vi "编码器线性位置测量_连续.vi"() -> ()   [LabVIEW 2013]
uses:
  <userlib>/ArtDAQ/_SubVI/ArtDAQ_CreateCILinEncoderChan.vi
  <userlib>/ArtDAQ/_SubVI/ArtDAQ_CfgSampClkTiming.vi
  <userlib>/ArtDAQ/_SubVI/ArtDAQ_Read Counter DBL NSamp.vi
panel:
  out "数据(米)":dbl[](array[numeric])
  in  "时钟源":string="/Dev1/PFI0"
  in  "每通道点数":i32=100
  in  "采样频率":dbl=1000.0 caption="采样速率" format="%0.6f"
  in  "Z索引相位":i32(ring)=10040 items=["A高B高"=10040, "A高B低"=10041, "A低B高"=10042, "A低B低"=10043]
  in  "解码类型":i32(ring)=10090 items=["X1"=10090, "X2"=10091, "X4"=10092, "TwoPulse"=10313]
  in  "脉冲间隔":dbl=0.0001
  in  "初始位置":dbl
  in  "Z索引值":dbl
  in  "启用Z索引":bool
  in  "Stop":bool
  in  "计数器":string="Dev1/ctr0"
  out "错误输出":errorcluster
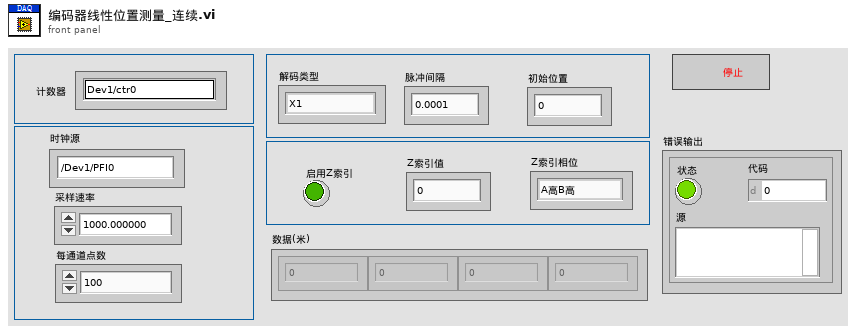
[diagram p1: front panel]
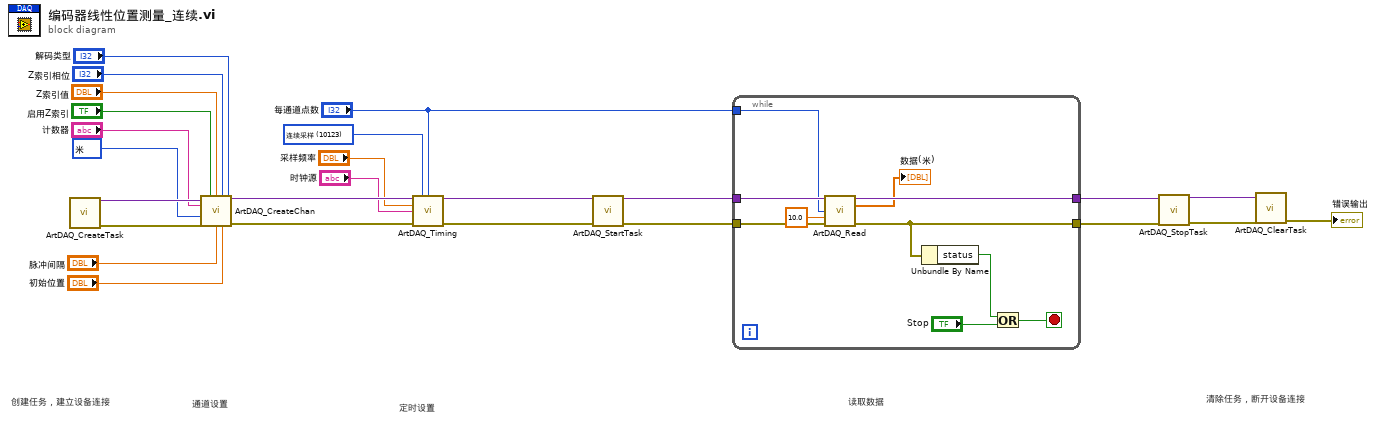
[diagram p0: block diagram]
diagram:
  w2 = 10123 items=["有限点采样"=10178, "连续采样"=10123] ("SampleMode")
  w11 = 10219 items=["米"=10219, "英寸"=10379, "时钟滴答"=10304, "来自自定义换算"=10065] ("单位")
  # "定时设置"
  # "清除任务，断开设备连接"
  # "读取数据"
  # "通道设置"
  # "创建任务，建立设备连接"
  n1 = call <userlib>:"ArtDAQ_CreateTask.vi"() -> ("任务句柄"=w25:variant, "错误输出"=w24:errorcluster)  [unwired: 14 in]
  n2 = call-poly <userlib>:"ArtDAQ_CreateChan.vi"("任务句柄"=w25, "启用Z索引"="启用Z索引", "Z索引值"="Z索引值", "Z索引相位"="Z索引相位", "计数器"="计数器", "解码类型"="解码类型", "单位"=w11, "错误输入"=w24, "脉冲间隔"="脉冲间隔", "初始位置"="初始位置") -> ("任务句柄"=w8:variant, "错误输出"=w5:errorcluster)  [unwired: 4 in]
  n3 = call-poly <userlib>:"ArtDAQ_Timing.vi"("任务句柄"=w8, "采样模式"=w2, "每通道采样数"="每通道点数", "采样率"="采样频率", "源"="时钟源", "错误输入"=w5) -> ("任务句柄"=w7:variant, "错误输出"=w6:errorcluster)  [unwired: 8 in]
  n4 = call <userlib>:"ArtDAQ_StartTask.vi"("任务句柄"=w7, "错误输入"=w6) -> ("任务句柄"=w14:variant, "错误输出"=w13:errorcluster)  [unwired: 12 in]
  n5 = while {
    tunnel: [w35] -> w22
    tunnel: [w34] -> w20
    tunnel: w14 -> [w33]
    tunnel: w13 -> [w32]
    tunnel: "每通道点数" -> [w26]
    stop <- w28 stop-if-true
    n6 = call-poly <userlib>:"ArtDAQ_Read.vi"("任务句柄"=w33, "每通道采样数"=w26, "超时s"=10.0 ("Timeout"), "错误输入"=w32) -> ("任务句柄"=w35:variant, "数据"=→"数据(米)":dbl[], "错误输出"=w34:errorcluster)  [unwired: 8 in, 1 out]
    n7 = Unbundle By Name(w34) -> ("status"=w30:bool)
    n8 = Or(x=w30, y="Stop") -> (x .or. y?=w28:bool)
  }
  n9 = call <userlib>:"ArtDAQ_StopTask.vi"("任务句柄"=w22, "错误输入"=w20) -> ("任务句柄"=w21:variant, "错误输出"=w19:errorcluster)  [unwired: 12 in]
  n10 = call <userlib>:"ArtDAQ_ClearTask.vi"("任务句柄"=w21, "错误输入"=w19) -> ("错误输出"=→"错误输出":errorcluster)  [unwired: 13 in]
